vi "test Send Message.vi"(8 "error in (no error)":errorcluster, 11 "TestCase in":refnum<class "Test Network Stream Transmission.lvclass">) -> (0 "error out":errorcluster, 3 "TestCase out":refnum<class "Test Network Stream Transmission.lvclass">)   [LabVIEW 2020, in "Test Network Stream Transmission.lvclass"]
uses:
  Test Network Stream Transmission.lvclass
  <vilib>/addons/_JKI Toolkits/VI Tester/TestCase.llb/TestCase.lvclass
  <vilib>/ActorFramework/LastAck/Last Ack.lvclass
  Source/Protocols/Network Stream Strategy/Network Stream Initiator/Network Stream Initiator.lvclass
  <vilib>/ActorFramework/Message/Message.lvclass
  Source/Abstract Classes/Cipher/Cipher.lvclass
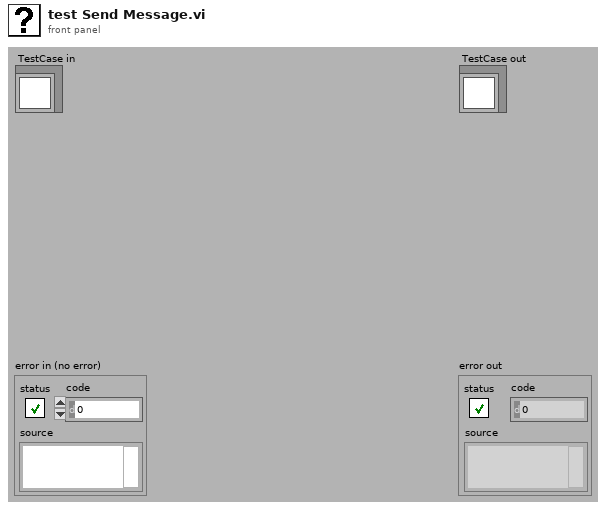
[diagram p1: front panel]
types:
  T1 = cluster{"Actor Framework.lvlib:Message.lvclass":refnum<class "Message.lvclass">, "priority":i32}
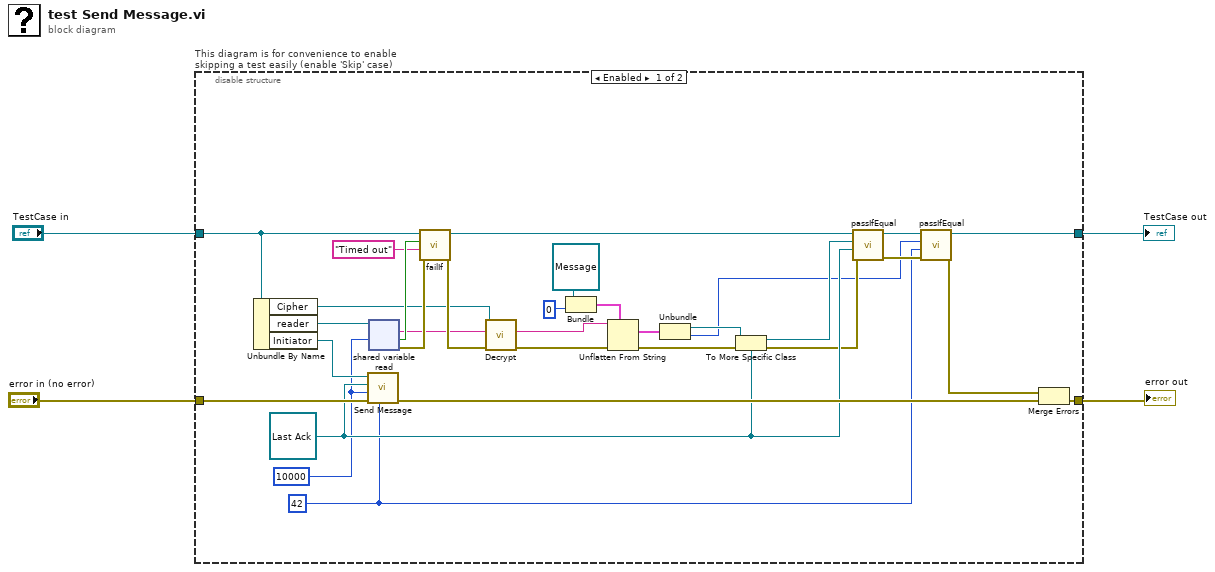
[diagram p0: block diagram]
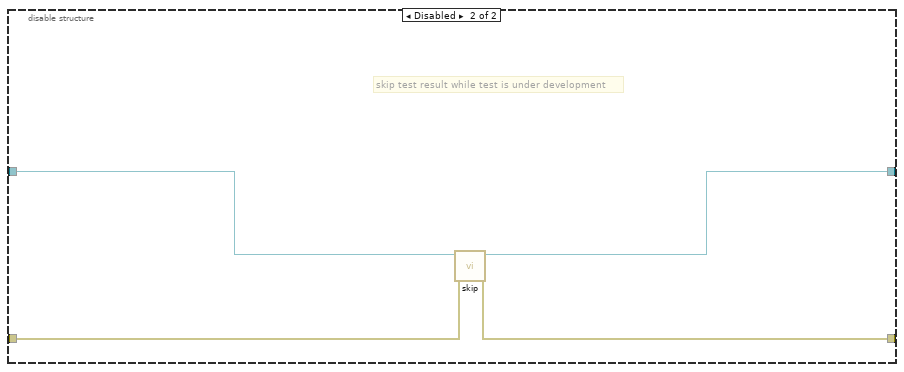
[diagram p2: hidden frame]
diagram:
  n1 = disable-structure "This diagram is for convenience to enable skipping a test easily (enable 'Skip' case)" shown="Enabled" {
    disable-tunnel: "TestCase in" -> [w26 w39]
    disable-tunnel: [w14 w37] -> w1
    disable-tunnel: [w20 w38] -> w3
    disable-tunnel: "error in (no error)" -> [w35 w36]
    frame Enabled {
      w10 = 42 ("priority")
      w27 = 10000 ("timeout ms (-1)")
      w28 = refnum<class "Last Ack.lvclass"> refnum ("Last Ack")
      n2 = Unbundle By Name(w26) -> ("Cipher"=w5:refnum<class "Cipher.lvclass">, "reader"=w32:refnum<k21>, "Initiator"=w33:refnum<class "Network Stream Initiator.lvclass">)
      n3 = call-dynamic "Send Message.vi"("priority"=w10, "error in (no error)"=w35, "timeout ms (-1)"=w27, "Message"=w28, "Network Stream in"=w33) -> ("error out"=w34:errorcluster)  [unwired: 5 in, 1 out]
      n4 = shared-variable-read(w32, w27) -> (w22:errorcluster, w24:bool, w7:string)  [unwired: 1 in, 1 out]
      n5 = call-dynamic "failIf.vi"("error in (no error)"=w22, "message (\"\")"="Timed out" ("message (\"\")"), "fail"=w24, "TestCase in"=w26) -> ("error out"=w8:errorcluster, "TestCase out"=w25:refnum<class "Test Network Stream Transmission.lvclass">)  [unwired: 6 in]
      n6 = call-dynamic "Decrypt.vi"("error in (no error)"=w8, "Ciphertext"=w7, "Cipher in"=w5) -> ("error out"=w9:errorcluster, "Plaintext"=w6:string)  [unwired: 6 in, 1 out]
      n7 = Bundle("Actor Framework.lvlib:Message.lvclass"=refnum<class "Message.lvclass"> refnum, "priority"=0) -> (w18:T1)  [unwired: 1 in]
      n8 = Unflatten From String(type=w18, binary string=w6, error in (no error)=w9) -> (value=w30:T1, error out=w31:errorcluster)  [unwired: 2 in, 1 out]
      n9 = Unbundle(w30) -> ("Actor Framework.lvlib:Message.lvclass"=w16:refnum<class "Message.lvclass">, "priority"=w11:i32)
      n10 = To More Specific Class(target class=w28, reference=w16, error in=w31) -> (specific class reference=w29:refnum<class "Last Ack.lvclass">, error out=w21:errorcluster)
      n11 = call-dynamic "passIfEqual.vi"("error in (no error)"=w21, "y"=w28, "x"=w29, "TestCase in"=w25) -> ("error out"=w13:errorcluster, "TestCase out"=w15:refnum<class "Test Network Stream Transmission.lvclass">)  [unwired: 6 in]
      n12 = call-dynamic "passIfEqual.vi"("error in (no error)"=w13, "y"=w10, "x"=w11, "TestCase in"=w15) -> ("error out"=w12:errorcluster, "TestCase out"=w14:refnum<class "Test Network Stream Transmission.lvclass">)  [unwired: 6 in]
      n13 = Merge Errors(w12, w34) -> (w20:errorcluster)
    }
    frame Disabled {
      # "skip test result while test is under development"
      n14 = call <vilib>:"skip.vi"("error in (no error)"=w36, "TestCase in"=w39) -> ("error out"=w38:errorcluster, "TestCase out"=w37:refnum<class "Test Network Stream Transmission.lvclass">)  [unwired: 8 in]
    }
  }
  "error out" <- w3
  "TestCase out" <- w1
